vi "Yscaling.vi"(7 "Scaling?":u16(ring) items=["Medium", "Large", "Small"], 10 "Plane Height (m)":dbl, 11 "?":cluster{"X":dbl, "Y":dbl, "Zpen":dbl}) -> (0 "Zpos Graph (nm)":T1, 3 "y scaled (m)":dbl, 4 "Position":cluster{"X":dbl, "Y":dbl, "Z pen":dbl, "Z":dbl})   [LabVIEW 2019]
uses:
  GlobalClicksHeight.vi
  <userlib>/HapticSTM/HapticSTM.lvlib
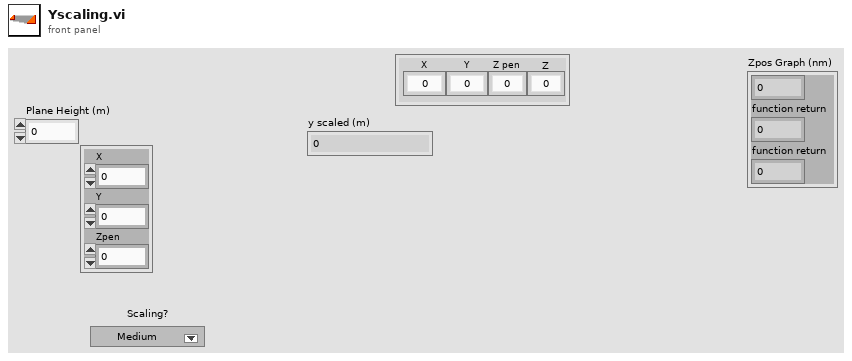
[diagram p1: front panel]
types:
  T1 = cluster{dbl, "function return":dbl, "function return":dbl}
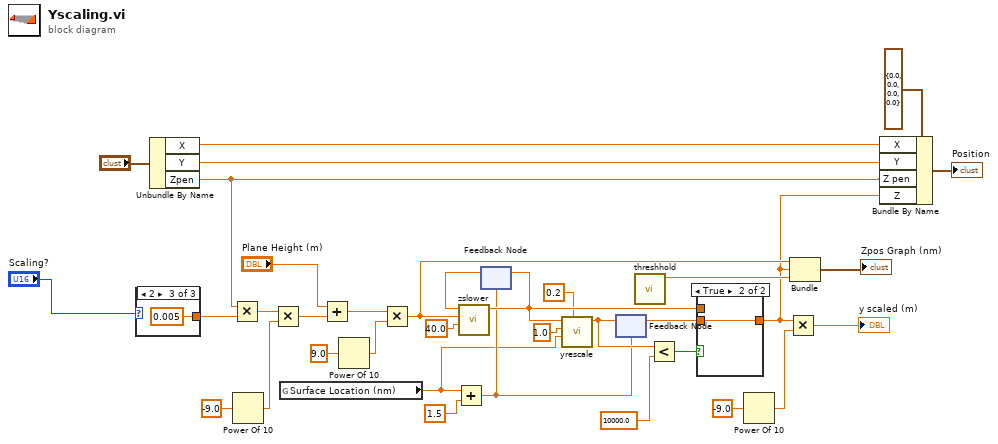
[diagram p0: block diagram]
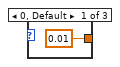
[diagram p2: hidden frame]
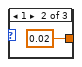
[diagram p3: hidden frame]
diagram:
  n1 = case shown="2" "Scaling?" {
    tunnel: [0.01 ("y") 0.02 ("y") 0.005 ("y")] -> w13
    frame 0, Default {
    }
    frame 1 {
    }
    frame 2 {
    }
  }
  n2 = Unbundle By Name("?") -> ("X"=w6:dbl, "Y"=w5:dbl, "Zpen"=w4:dbl)
  n3 = Multiply(x=w4, y=w13) -> (x*y=w31:dbl)
  n4 = Power Of 10(x=-9.0) -> (10^x=w30:dbl)
  n5 = Multiply(x=w31, y=w30) -> (x*y=w32:dbl)
  n6 = global read "GlobalClicksHeight.vi" "Surface Location (nm)"() -> (w9:dbl)
  n7 = Add(x="Plane Height (m)", y=w32) -> (x+y=w35:dbl)
  n8 = Power Of 10(x=9.0) -> (10^x=w34:dbl)
  n9 = Multiply(x=w35, y=w34) -> (x*y=w18:dbl)
  n10 = Add(x=w9, y=1.5) -> (x+y=w14:dbl)
  n11 = feedback #1(w14) -> (w20:dbl)
  n12 = call <userlib>:"zslower.vi"("maxvel"=40.0, "labview_zpos_write"=w18, "nanonis_zpos_read"=w20) -> ("function return"=w16:dbl)  [unwired: 8 in]
  n13 = feedback-in #1(w16) -> ()
  n14 = call <userlib>:"yrescale.vi"("plunge"=0.2, "surf"=w9, "scalingfactor"=1.0, "ylabview"=w16) -> ("function return"=w17:dbl)  [unwired: 7 in]
  n15 = feedback-in #2(w17) -> ()
  n16 = feedback #2(w14) -> (w22:dbl)
  n17 = call <userlib>:"threshhold.vi"() -> ("function return"=w12:dbl)  [unwired: 11 in]
  n18 = Less?(x=w17, y=10000.0) -> (x < y?=w23:bool)
  n19 = case shown="True" w23 {
    tunnel: [w39 w40] -> w1
    tunnel: w22 -> [_ w40]
    tunnel: w16 -> [w39 _]
    frame False {
    }
    frame True {
    }
  }
  n20 = Power Of 10(x=-9.0) -> (10^x=w26:dbl)
  n21 = Multiply(x=w1, y=w26) -> (x*y=→"y scaled (m)":dbl)
  n22 = Bundle(w18, "function return"=w1, "function return"=w12) -> (→"Zpos Graph (nm)":T1)  [unwired: 1 in]
  n23 = Bundle By Name(cluster=cluster{"X":dbl, "Y":dbl, "Z pen":dbl, "Z":dbl} {"X"=0.0, "Y"=0.0, "Z pen"=0.0, "Z"=0.0} ("Position"), "X"=w6, "Y"=w5, "Z pen"=w4, "Z"=w1) -> (→"Position":cluster{"X":dbl, "Y":dbl, "Z pen":dbl, "Z":dbl})
